vi "Parse Error XML.vi"(9 "Code Tag Value":string, 10 "Error XML":string) -> (0 "Unknown Error":bool, 1 "Error Description Override":string, 2 "Error Code":i32, 3 "Warning":bool)   [LabVIEW 2015, in "NI_Azure_Queue.lvlib"]
uses:
  NI_Azure_Queue.lvlib
  Core/NI_Azure_Core.lvlib
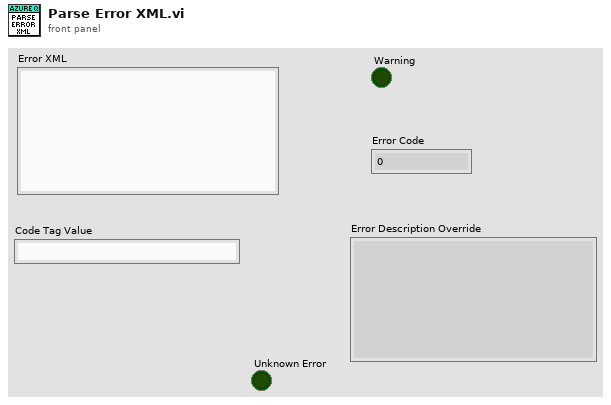
[diagram p1: front panel]
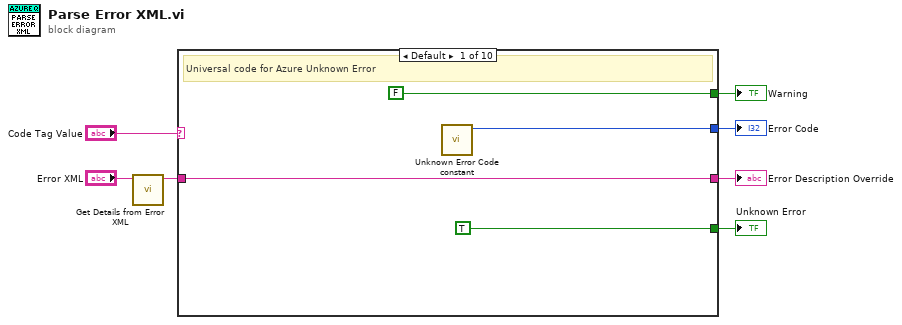
[diagram p0: block diagram]
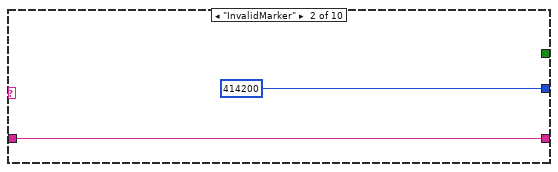
[diagram p2: hidden frame]
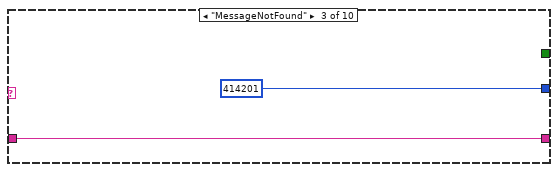
[diagram p3: hidden frame]
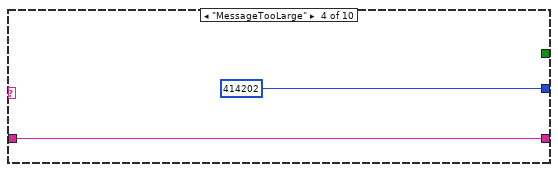
[diagram p4: hidden frame]
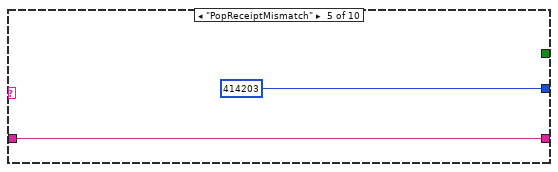
[diagram p5: hidden frame]
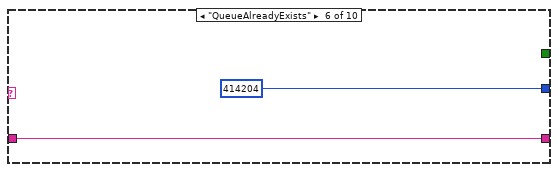
[diagram p6: hidden frame]
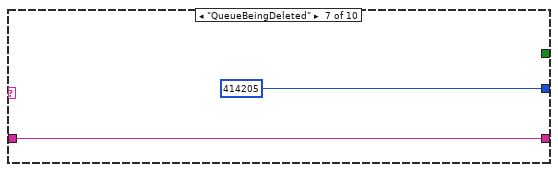
[diagram p7: hidden frame]
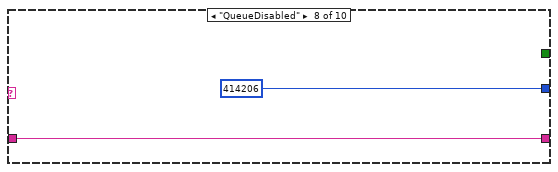
[diagram p8: hidden frame]
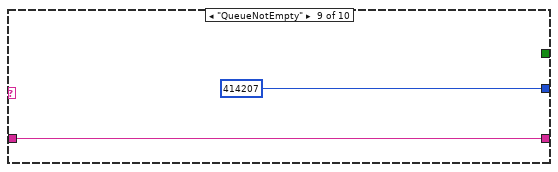
[diagram p9: hidden frame]
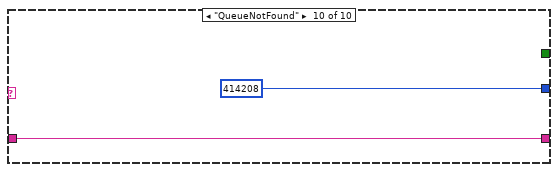
[diagram p10: hidden frame]
diagram:
  n1 = call "Get Details from Error XML.vi"("Error XML"="Error XML") -> ("Details"=w1:string)  [unwired: 10 in]
  n2 = case shown="Default" "Code Tag Value" {
    tunnel: [w10 414200 414201 414202 414203 414204 414205 414206 414207 414208] -> w5
    tunnel: [FALSE _ _ _ _ _ _ _ _ _] -> w6
    tunnel: w1 -> [w9 w12 w14 w16 w18 w20 w22 w24 w26 w28]
    tunnel: [w9 w12 w14 w16 w18 w20 w22 w24 w26 w28] -> w4
    tunnel: [TRUE _ _ _ _ _ _ _ _ _] -> w3
    frame Default {
      # "Universal code for Azure Unknown Error"
      n3 = call "Unknown Error Code constant.vi"() -> ("Azure Unknown Error Code value"=w10:i32)  [unwired: 11 in]
    }
    frame "InvalidMarker" {
    }
    frame "MessageNotFound" {
    }
    frame "MessageTooLarge" {
    }
    frame "PopReceiptMismatch" {
    }
    frame "QueueAlreadyExists" {
    }
    frame "QueueBeingDeleted" {
    }
    frame "QueueDisabled" {
    }
    frame "QueueNotEmpty" {
    }
    frame "QueueNotFound" {
    }
  }
  "Error Description Override" <- w4
  "Warning" <- w6
  "Error Code" <- w5
  "Unknown Error" <- w3
